vi "Execute OutrTerm Handle.vi"(6 "Menu Item Tag Suffix":string, 8 "错误输入（无错误）":errorcluster, 11 "外部接线端输入":refnum<vi>) -> (0 "错误输出":errorcluster)   [LabVIEW 2020]
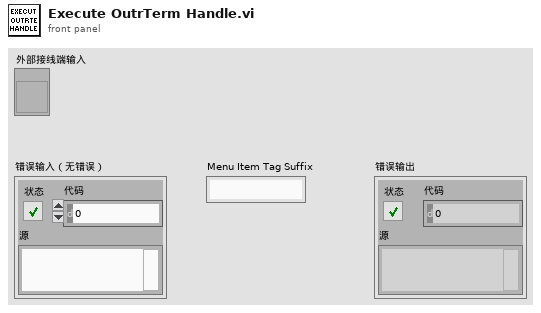
[diagram p1: front panel]
types:
  T1 = typedef "LVRectTypeDef.ctl" = cluster{"Left":i16, "Top":i16, "Right":i16, "Bottom":i16}
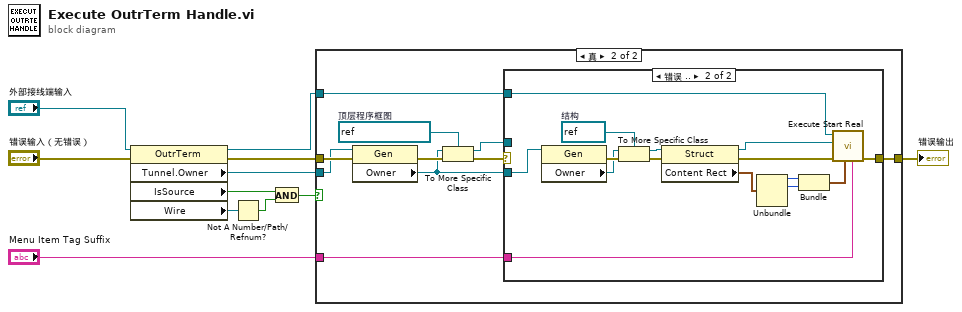
[diagram p0: block diagram]
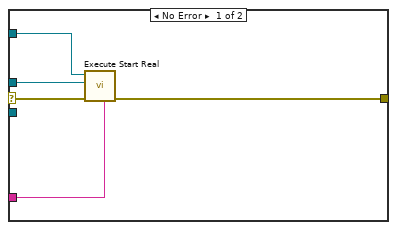
[diagram p3: hidden frame]
diagram:
  n1 = property class="OutrTerm"(reference="外部接线端输入", error in="错误输入（无错误）") -> (reference out=w8:refnum<vi>, error out=w11:errorcluster, "Tunnel.Owner"=w9:refnum<vi>, "IsSource"=w4:bool, "Wire"=w3:refnum<vi>)
  n2 = Not A Number/Path/Refnum?(number/path/refnum=w3) -> (NaN/Path/Refnum?=w1:bool)
  n3 = And(x=w4, y=w1) -> (x .and. y?=w2:bool)
  n4 = case shown="真" w2 {
    tunnel: w8 -> [_ w19]
    tunnel: w9 -> [_ w13]
    tunnel: "Menu Item Tag Suffix" -> [_ w18]
    tunnel: w11 -> [w12 w17]
    tunnel: [w12 w14] -> w5
    frame False {
    }
    frame True {
      w22 = refnum<vi> refnum  # 顶层程序框图
      n5 = property class="Gen"(reference=w13, error in=w17) -> (error out=w16:errorcluster, "Owner"=w15:refnum<vi>)  [unwired: 1 out]
      n6 = To More Specific Class(target class=w22, reference=w15, error in=w16) -> (specific class reference=w20:refnum<vi>, error out=w21:errorcluster)
      n7 = case shown="错误 .." w21 {
        selector: w21 -> [w27 _]
        tunnel: w20 -> [w26 _]
        tunnel: w19 -> [w25 w35]
        tunnel: w18 -> [w23 w29]
        tunnel: w15 -> [_ w32]
        tunnel: [w24 w30] -> w14
        frame No Error {
          n8 = call "Execute Start Real.vi"("Menu Item Tag Suffix"=w23, "错误输入（无错误）"=w27, "所有者引用句柄"=w26, "接线端输入"=w25) -> ("错误输出"=w24:errorcluster)  [unwired: 7 in]
        }
        frame Error {
          w42 = refnum<vi> refnum  # 结构
          n9 = property class="Gen"(reference=w32) -> (error out=w33:errorcluster, "Owner"=w31:refnum<vi>)  [unwired: 1 in, 1 out]
          n10 = To More Specific Class(target class=w42, reference=w31, error in=w33) -> (specific class reference=w40:refnum<vi>, error out=w41:errorcluster)
          n11 = property class="Struct"(reference=w40, error in=w41) -> (reference out=w34:refnum<vi>, error out=w36:errorcluster, "Content Rect"=w39:T1)
          n12 = Unbundle(w39) -> ("Left"=w38:i16, "Top"=w37:i16)  [unwired: 2 out]
          n13 = Bundle("Left"=w38, "Top"=w37) -> (w28:cluster{"Left":i16, "Top":i16})  [unwired: 1 in]
          n14 = call "Execute Start Real.vi"("Menu Item Tag Suffix"=w29, "相对位置原点"=w28, "错误输入（无错误）"=w36, "所有者引用句柄"=w34, "接线端输入"=w35) -> ("错误输出"=w30:errorcluster)  [unwired: 6 in]
        }
      }
    }
  }
  "错误输出" <- w5
